vi "Stop DI.vi"(0 "reference in":refnum<class "DI.lvclass">, 5 "error in (no error)":errorcluster) -> (14 "reference out":refnum<class "DI.lvclass">, 19 "error out":errorcluster)   [LabVIEW 2017, in "DI.lvclass"]
uses:
  DI.lvclass
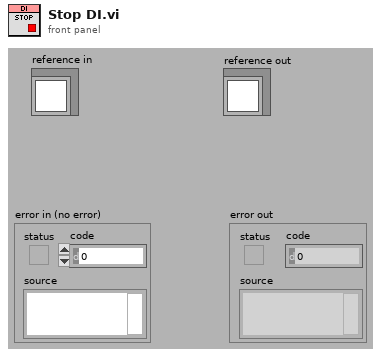
[diagram p1: front panel]
types:
  T1 = typedef "DI.lvclass/ObjectAttributes.ctl" = cluster{"DI Task":refnum<k21>, "DI Status":bool[], "DI Module Names (NI-Max Name)":string[], "Number of Channels Per DI Module":i32[], "Number of DI Modules":u32, "Number of Total DI Channels":u32, "DI On/Off Status":bool, "DO VI Reference":refnum<vi>}
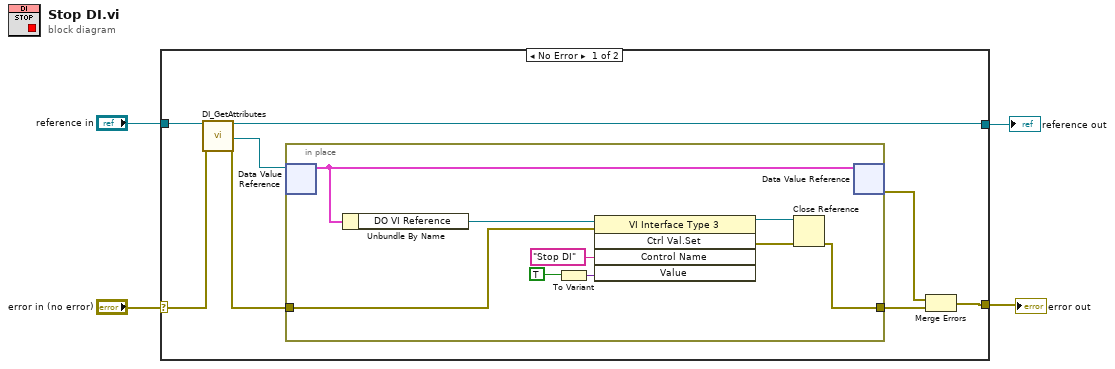
[diagram p0: block diagram]
diagram:
  n1 = case shown="No Error" "error in (no error)" {
    selector: "error in (no error)" -> [w11 w23]
    tunnel: [w8 w23] -> w3
    tunnel: [w9 w22] -> w1
    tunnel: "reference in" -> [w12 w22]
    frame No Error {
      n2 = call "DI_GetAttributes.vi"("reference in"=w12, "error in (no error)"=w11) -> ("reference out"=w9:refnum<class "DI.lvclass">, "DataRef"=w7:refnum<data-value>, "error out"=w6:errorcluster)  [unwired: 14 in, 1 out]
      n3 = in-place {
        in-place-border: w6 -> [w18]
        in-place-border: [w17] -> w5
        n4 = in-place-dvr #1(w7) -> (w16:T1)  [unwired: 1 out]
        n5 = Unbundle By Name(w16) -> ("DO VI Reference"=w21:refnum<vi>)
        n6 = To Variant(anything=TRUE) -> (Variant=w14:variant)
        n7 = invoke class="VI Interface Type 3" method="Ctrl Val.Set"(reference=w21, error in=w18, "Control Name"="Stop DI", "Value"=w14) -> (reference out=w20:refnum<vi>, error out=w19:errorcluster)  [unwired: 1 in, 3 out]
        n8 = Close Reference(reference=w20, error in (no error)=w19) -> (error out=w17:errorcluster)
        n9 = in-place-dvr #1(w16) -> (w10:errorcluster)  [unwired: 1 out]
      }
      n10 = Merge Errors(w10, w5) -> (w8:errorcluster)
    }
    frame Error {
    }
  }
  "error out" <- w3
  "reference out" <- w1
